vi "vision data cache.vi"(2 "State In":enum16{"Tracking", "Locked", "Out of Range"}(ring), 3 "Data Input":T1, 4 "Menu (Get)":enum16{"Get", "Set"}(ring)) -> (0 "State Out":enum16{"Tracking", "Locked", "Out of Range"}(ring), 1 "Data Output":T1)   [LabVIEW 2011]
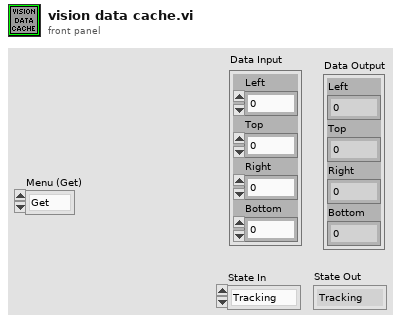
[diagram p1: front panel]
types:
  T1 = cluster{"Left":i32, "Top":i32, "Right":i32, "Bottom":i32}
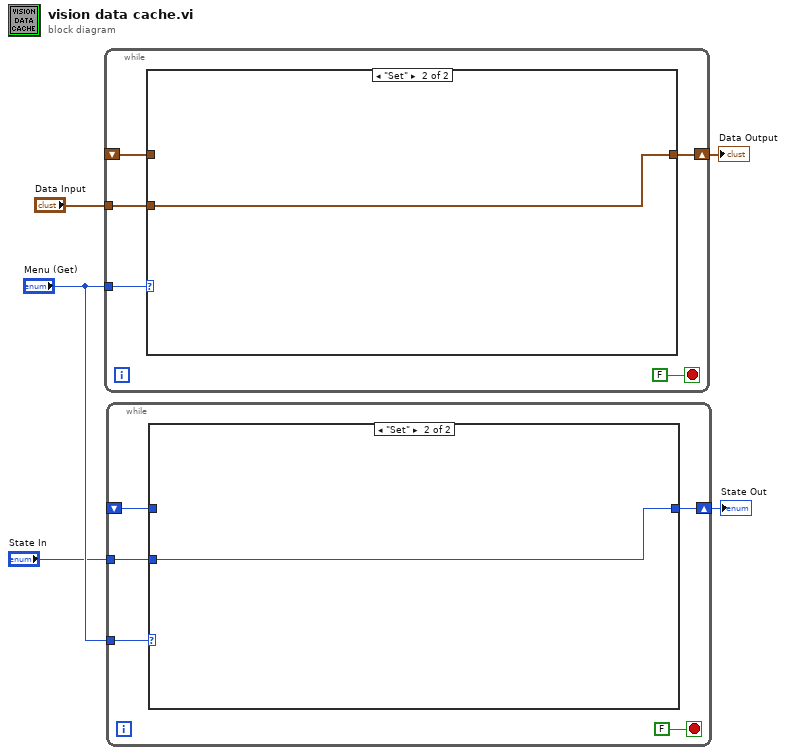
[diagram p0: block diagram]
diagram:
  n1 = while {
    shift-right: [w8] -> w4
    shift-left: _ -> [w6]
    tunnel: "Data Input" -> [w7]
    tunnel: "Menu (Get)" -> [w9]
    stop <- FALSE stop-if-true
    n2 = case shown="\"Set\"" w9 {
      tunnel: [w11 w12] -> w8
      tunnel: w7 -> [_ w12]
      tunnel: w6 -> [w11 _]
      frame "Get", Default {
      }
      frame "Set" {
      }
    }
  }
  "Data Output" <- w4
  n3 = while {
    shift-right: [w15] -> w1
    shift-left: _ -> [w13]
    tunnel: "State In" -> [w14]
    tunnel: "Menu (Get)" -> [w16]
    stop <- FALSE stop-if-true
    n4 = case shown="\"Set\"" w16 {
      tunnel: [w18 w19] -> w15
      tunnel: w14 -> [_ w19]
      tunnel: w13 -> [w18 _]
      frame "Get", Default {
      }
      frame "Set" {
      }
    }
  }
  "State Out" <- w1
